vi "Create queue.vi"(8 "error in (no error)":errorcluster) -> (0 "error out":errorcluster, 3 "Transporter out":refnum<class "Transporter.lvclass">)   [LabVIEW 2021, in "Msn Trasnsportation Library 1.lvlib" / "Transporter.lvclass"]
uses:
  Transporter.lvclass
  Message.lvclass
  Transporter.lvclass/Transporter.ctl
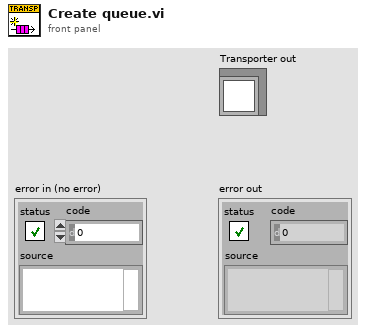
[diagram p1: front panel]
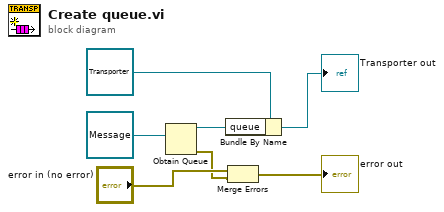
[diagram p0: block diagram]
diagram:
  n1 = Obtain Queue(element data type=refnum<class "Message.lvclass"> refnum ("Msn Trasnsportation Library 1.lvlib:MessagE")) -> (queue out=w4:refnum<queue>, error out=w1:errorcluster)  [unwired: 4 in, 1 out]
  n2 = Bundle By Name(cluster=refnum<class "Transporter.lvclass"> refnum ("Transporter in"), "queue"=w4) -> (→"Transporter out":refnum<class "Transporter.lvclass">)
  n3 = Merge Errors("error in (no error)", w1) -> (→"error out":errorcluster)
